vi "mqttClient_Viewer.vi"() -> ()   [LabVIEW 2019]
uses:
  <vilib>/LabVIEW Open Source Project/OpenSerializer JKI JSON/Serializer.JSON.lvclass
  C:/Program Files (x86)/National Instruments/LabVIEW 2019/vi.lib/LabVIEW Open Source Project/OpenSerializer/Serializer/Serializer.lvclass
  DUT/state -- cluster.ctl
  <vilib>/LabVIEW Open Source Project/MQTT Connection/MQTT_Base/Base Class/MQTT_Base.lvclass/MQTT_Base.ctl
  <vilib>/LabVIEW Open Source Project/MQTT Client/Client class/Client.lvclass/Client.ctl
  DUT/target -- cluster.ctl
  <vilib>/LabVIEW Open Source Project/MQTT Control Packets/Control Packets/ControlPacket/QualityOfService -- enum.ctl
  <vilib>/LabVIEW Open Source Project/MQTT Control Packets/Control Packets/ControlPacket/ControlPacket.lvclass/ControlPacket.ctl
  <vilib>/LabVIEW Open Source Project/MQTT Control Packets/Control Packets/CONNECT/ConnectFlags -- cluster.ctl
  <vilib>/LabVIEW Open Source Project/MQTT TCP Connection/MQTT_TCP/Connection/TCPConnection.lvclass
  C:/Program Files (x86)/National Instruments/LabVIEW 2019/vi.lib/LabVIEW Open Source Project/MQTT Connection/MQTT_Connection/Connection/Connection.lvclass
  <vilib>/LabVIEW Open Source Project/MQTT Client/Client class/Client.lvclass
  C:/Program Files (x86)/National Instruments/LabVIEW 2019/vi.lib/LabVIEW Open Source Project/MQTT Connection/MQTT_Base/Base Class/MQTT_Base.lvclass
  <vilib>/LabVIEW Open Source Project/OpenSerializer/Serializer.FlattenedString/Serializer.FlattenedString.lvclass
  <vilib>/LabVIEW Open Source Project/MQTT Control Packets/Control Packets/PUBLISH/PUBLISH.lvclass
  C:/Program Files (x86)/National Instruments/LabVIEW 2019/vi.lib/LabVIEW Open Source Project/MQTT Control Packets/Control Packets/ControlPacket/ControlPacket.lvclass
  <vilib>/LabVIEW Open Source Project/OpenSerializer/Serializer/Serializer.lvclass
  <vilib>/LabVIEW Open Source Project/MQTT Connection/MQTT_Base/Base Class/MQTT_Base.lvclass
  <vilib>/LabVIEW Open Source Project/MQTT Control Packets/Control Packets/CONNECT/CONNECT.lvclass
  <vilib>/LabVIEW Open Source Project/MQTT Control Packets/Control Packets/ControlPacket/ControlPacket.lvclass
panel:
  out "Incoming Messages":string
  in  "Connection":bool
  out "last error":errorcluster
  in  "setpoint":dbl format="%.1g"
  in  "enabled":bool
  out "Waveform Chart":cluster{"setpoint":dbl, "measured":dbl}(graph)
  # "Native LabVIEW MQTT Client (View)"
  # "G Open Source Project for LabVIEW\nhttps://github.com/LabVIEW-Open-Source/MQTT-Client"
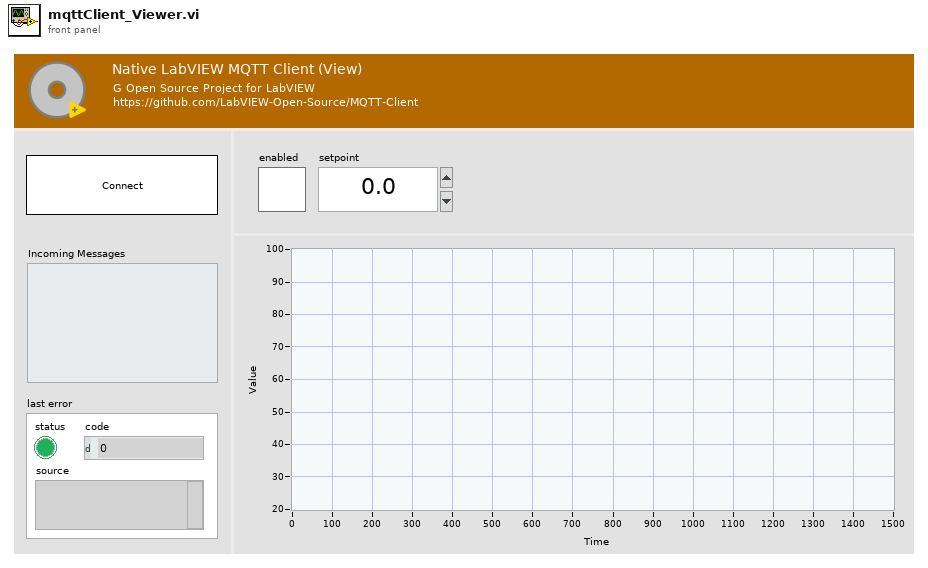
[diagram p1: front panel]
types:
  T1 = typedef "state -- cluster.ctl" = cluster{"enabled":bool, "setpoint":dbl, "measured":dbl}
  T2 = typedef "MQTT Client.lvlib/Client.lvclass/Public Events -- cluster.ctl" = cluster{"Connection Status":refnum<user-event>, "Connected":refnum<user-event>, "Application Message":refnum<user-event>}
  T3 = typedef "MQTT Base.lvlib/MQTT_Base.lvclass/Public Events -- cluster.ctl" = cluster{"Stop Event":refnum<user-event>, "Error Event":refnum<user-event>, "Inbound Message":refnum<user-event>}
  T4 = typedef "MQTT_Control_Packets.lvlib/ControlPacket.lvclass/QualityOfService -- enum.ctl" = enum16{"0 (At Most Once)", "1 (At Least Once)", "2 (Exactly Once)"}
  T5 = typedef "MQTT_Control_Packets.lvlib/CONNECT.lvclass/ConnectFlags -- cluster.ctl" = cluster{"Reserved":bool, "Clean Session":bool, "Will Flag":bool, "Will QoS 1":bool, "Will QoS 2":bool, "Will Retain":bool, "Password Flag":bool, "User Name Flag":bool}
  T6 = typedef "target -- cluster.ctl" = cluster{"enabled":bool, "setpoint":dbl}
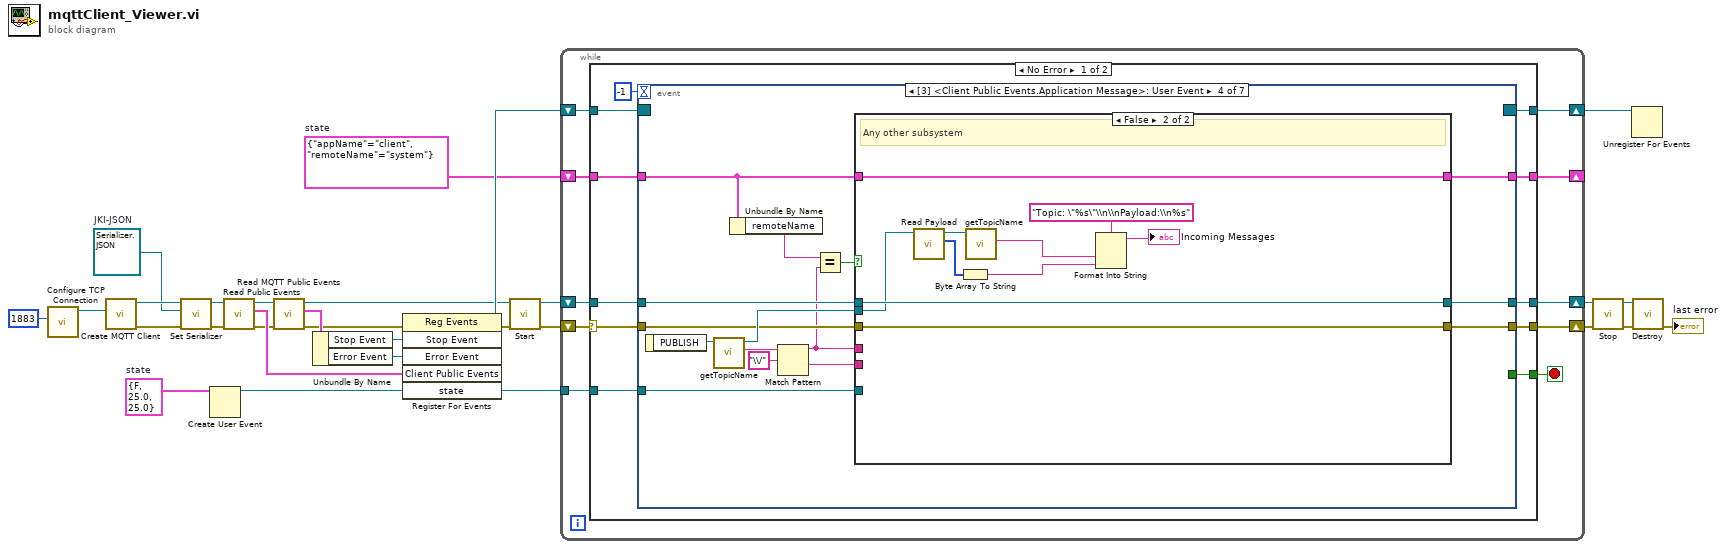
[diagram p0: block diagram]
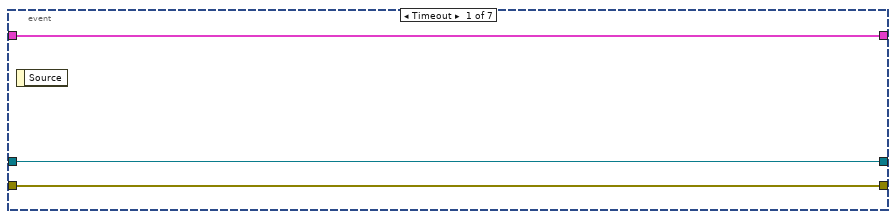
[diagram p2: hidden frame]
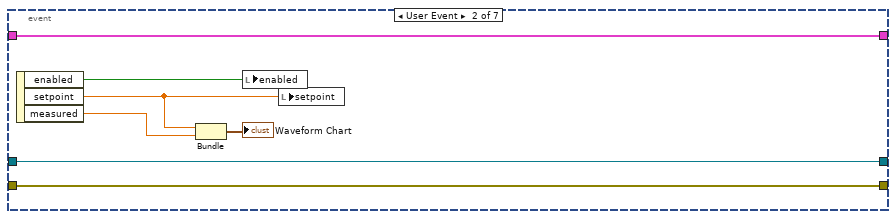
[diagram p3: hidden frame]
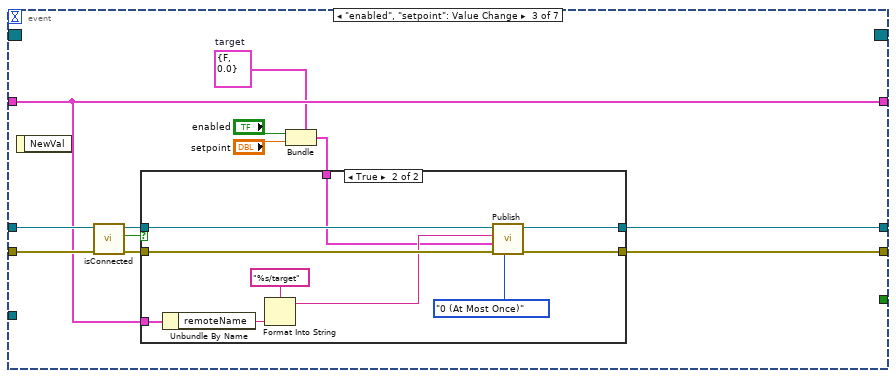
[diagram p4: hidden frame]
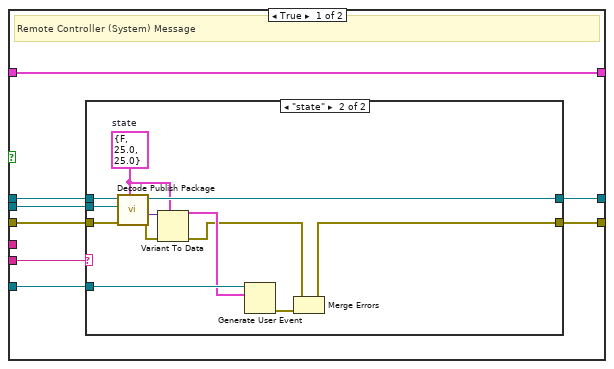
[diagram p6: hidden frame]
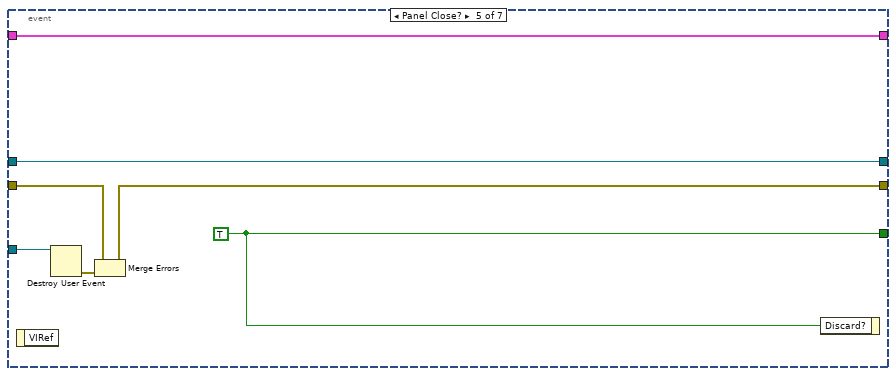
[diagram p8: hidden frame]
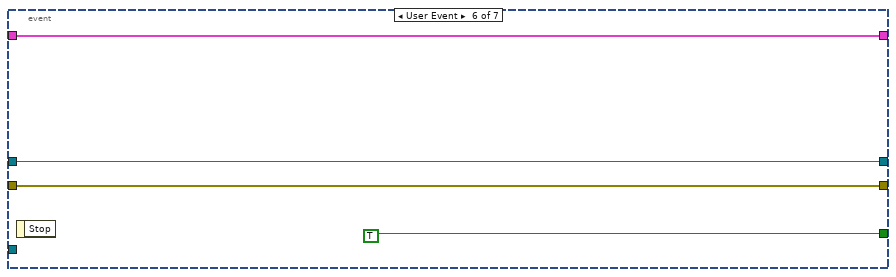
[diagram p9: hidden frame]
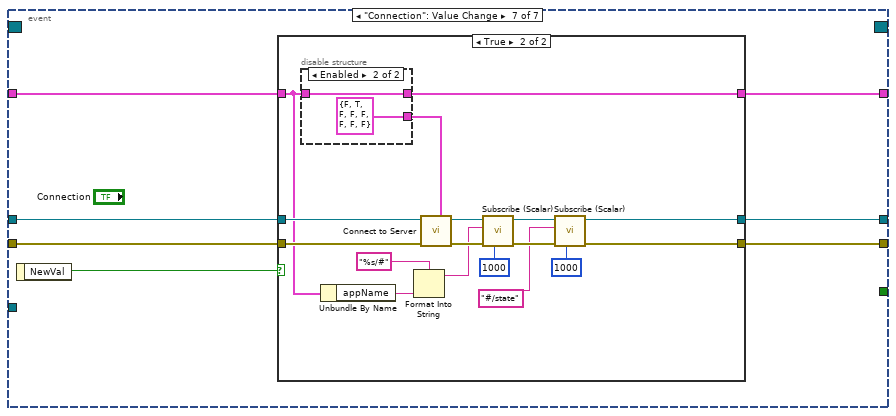
[diagram p10: hidden frame]
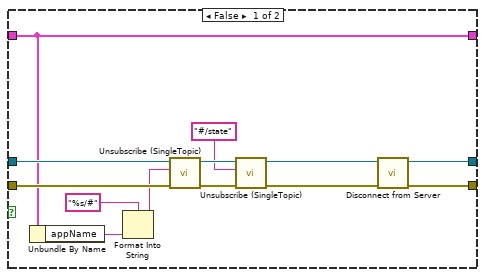
[diagram p11: hidden frame]
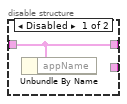
[diagram p12: hidden frame]
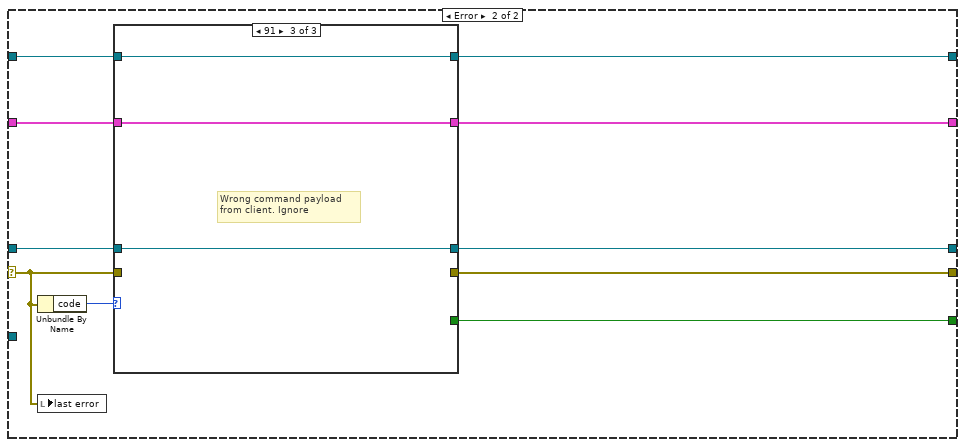
[diagram p13: hidden frame]
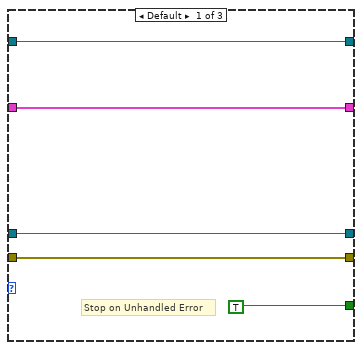
[diagram p14: hidden frame]
diagram:
  w2 = T1 {"enabled"=FALSE, "setpoint"=25.0, "measured"=25.0}  # state
  w3 = cluster{"appName":string, "remoteName":string} {"appName"="client", "remoteName"="system"}  # state
  w6 = refnum<class "Serializer.JSON.lvclass"> refnum  # JKI-JSON
  n1 = call <vilib>:"Configure TCP Connection.vi"("remote port (80)"=u16 1883) -> ("TCPConnection"=w11:refnum<class "TCPConnection.lvclass">)  [unwired: 9 in, 1 out]
  n2 = call <vilib>:"Create MQTT Client.vi"("Connection Configuration"=w11) -> ("error out"=w8:errorcluster, "Client out"=w10:refnum<class "Client.lvclass">)  [unwired: 9 in]
  n3 = call <vilib>:"Set Serializer.vi"("error in (no error)"=w8, "Serializer (default: Flattened String)"=w6, "MQTT_Base"=w10) -> ("error out"=w7:errorcluster, "MQTT_Base out"=w9:refnum<class "Client.lvclass">)  [unwired: 7 in]
  n4 = Create User Event(user event datatype=w2) -> (user event=w1:refnum<user-event>)  [unwired: 1 in, 1 out]
  n5 = call <vilib>:"Read Public Events.vi"("error in (no error)"=w7, "Client in"=w9) -> ("error out"=w13:errorcluster, "Client Public Events"=w15:T2, "Client out"=w12:refnum<class "Client.lvclass">)  [unwired: 7 in]
  n6 = call <vilib>:"Read MQTT Public Events.vi"("error in (no error)"=w13, "MQTT_Base in"=w12) -> ("error out"=w14:errorcluster, "MQTT Public Events"=w22:T3, "MQTT_Base out"=w17:refnum<class "Client.lvclass">)  [unwired: 7 in]
  n7 = Unbundle By Name(w22) -> ("Stop Event"=w20:refnum<user-event>, "Error Event"=w21:refnum<user-event>)
  n8 = register-events(error in=w14, w20, w21, w15, w1) -> (reference out=w18:refnum<event-registration>, error out=w16:errorcluster)  [unwired: 1 in]
  n9 = call <vilib>:"Start.vi"("error in (no error)"=w16, "MQTT_Base in"=w17) -> ("error out"=w4:errorcluster, "MQTT_Base out"=w5:refnum<class "Client.lvclass">)  [unwired: 7 in, 1 out]
  n10 = while {
    shift-right: [w37] -> w19
    shift-left: w18 -> [w38]
    shift-right: [w34] -> w24
    shift-left: w5 -> [w35]
    shift-right: [w36] -> w26
    shift-left: w4 -> [w32]
    shift-right: [w30] -> _
    shift-left: w3 -> [w31]
    tunnel: w1 -> [w29]
    stop <- w33 stop-if-true
    n11 = case shown="No Error" w32 {
      selector: w32 -> [w42 w185]
      tunnel: w38 -> [w49 w184]
      tunnel: [w48 w183] -> w37
      tunnel: [w47 w188] -> w36
      tunnel: w35 -> [w45 w189]
      tunnel: [w44 w191] -> w34
      tunnel: [w43 w187] -> w33
      tunnel: w31 -> [w41 w186]
      tunnel: [w40 w182] -> w30
      tunnel: w29 -> [w39 _]
      frame No Error {
        n12 = event shown="[3] <Client Public Events.Application Message>: User Event" {
          selector: w49 -> [_ _ _ _ _ _ _]
          dyn-events: [_ _ _ _ _ _ _] -> w48
          timeout: -1 -> [_ _ _ _ _ _ _]
          tunnel: w42 -> [w50 w57 w67 w95 w131 w141 w144]
          tunnel: [w50 w57 w61 w93 w132 w141 w145] -> w47
          tunnel: [_ _ _ _ w137 TRUE _] -> w43
          tunnel: w45 -> [w51 w58 w68 w96 w136 w139 w148]
          tunnel: [w51 w58 w62 w94 w136 w139 w146] -> w44
          tunnel: w41 -> [w52 w59 w66 w87 w135 w138 w142]
          tunnel: [w52 w59 w66 w92 w135 w138 w143] -> w40
          tunnel: w39 -> [_ _ _ w84 w134 _ _]
          event Timeout {
            n13 = event-data() -> ()  [unwired: 1 in, 1 out]
          }
          event User Event {
            n14 = event-data() -> ("enabled"=w55:bool, "setpoint"=w53:dbl, "measured"=w54:dbl)  [unwired: 1 in]
            n15 = Bundle("setpoint"=w53, "measured"=w54) -> (→"Waveform Chart":cluster{"setpoint":dbl, "measured":dbl})  [unwired: 1 in]
            n16 = local write "enabled"(w55) -> ()
            n17 = local write "setpoint"(w53) -> ()
          }
          event "enabled", "setpoint": Value Change {
            w60 = T6 {"enabled"=FALSE, "setpoint"=0.0}  # target
            n18 = event-data() -> ()  [unwired: 1 in, 1 out]
            n19 = call <vilib>:"isConnected.vi"("error in (no error)"=w67, "Client in"=w68) -> ("error out"=w71:errorcluster, "connected"=w69:bool, "Client out"=w70:refnum<class "Client.lvclass">)  [unwired: 7 in]
            n20 = Bundle(cluster=w60, "enabled"="enabled", "setpoint"="setpoint") -> (w63:T6)
            n21 = case shown="True" w69 {
              tunnel: [w73 w82] -> w62
              tunnel: [w72 w80] -> w61
              tunnel: w70 -> [w73 w83]
              tunnel: w71 -> [w72 w81]
              tunnel: w66 -> [_ w75]
              tunnel: w63 -> [_ w74]
              frame False {
              }
              frame True {
                n22 = Unbundle By Name(w75) -> ("remoteName"=w78:string)
                n23 = Format Into String(format string="%s/target" ("Topic Name (empty: Payload name)"), w78) -> (resulting string=w76:string)  [unwired: 2 in, 1 out]
                n24 = call <vilib>:"Publish.vi"("QoS"=QualityOfService_--_enum."0 (At Most Once)", "error in (no error)"=w81, "Payload"=w74, "Topic Name (empty: Payload name)"=w76, "Client in"=w83) -> ("error out"=w80:errorcluster, "Client out"=w82:refnum<class "Client.lvclass">)  [unwired: 4 in, 1 out]
              }
            }
          }
          event User Event {
            n25 = event-data() -> ("PUBLISH"=w98:refnum<class "PUBLISH.lvclass">)  [unwired: 1 in]
            n26 = call <vilib>:"getTopicName.vi"("PUBLISH in"=w98) -> ("Topic"=w90:string, "PUBLISH out"=w97:refnum<class "PUBLISH.lvclass">)  [unwired: 8 in, 1 out]
            n27 = Unbundle By Name(w87) -> ("remoteName"=w88:string)
            n28 = Match Pattern(string=w90, regular expression="\\/") -> (before substring=w86:string, after substring=w89:string)  [unwired: 1 in, 2 out]
            n29 = Equal?(x=w88, y=w86) -> (x = y?=w85:bool)
            n30 = case shown="False" w85 {
              tunnel: w97 -> [w103 w121]
              tunnel: w96 -> [w105 w129]
              tunnel: w95 -> [w104 w128]
              tunnel: [w102 w129] -> w94
              tunnel: [w101 w128] -> w93
              tunnel: w87 -> [w106 w130]
              tunnel: [w106 w130] -> w92
              tunnel: w89 -> [w100 _]
              tunnel: w86 -> [_ _]
              tunnel: w84 -> [w99 _]
              frame True {
                # "Remote Controller (System) Message"
                n31 = case shown="\"state\"" w100 {
                  tunnel: w105 -> [w108 w120]
                  tunnel: w104 -> [w107 w119]
                  tunnel: w103 -> [_ w118]
                  tunnel: [w108 w117] -> w102
                  tunnel: [w107 w109] -> w101
                  tunnel: w99 -> [_ w113]
                  frame Default {
                  }
                  frame "state" {
                    w114 = T1 {"enabled"=FALSE, "setpoint"=25.0, "measured"=25.0}  # state
                    n32 = call <vilib>:"Decode Publish Package.vi"("Type"=w114, "error in (no error)"=w119, "PUBLISH"=w118, "MQTT_Base in"=w120) -> ("error out"=w115:errorcluster, "Payload"=w116:variant, "MQTT_Base out"=w117:refnum<class "Client.lvclass">)  [unwired: 4 in, 1 out]
                    n33 = Variant To Data(error in=w115, type=w114, Variant=w116) -> (data=w112:T1, error out=w110:errorcluster)
                    n34 = Generate User Event(user event=w113, event data cluster=w112) -> (error out=w111:errorcluster)  [unwired: 2 in, 1 out]
                    n35 = Merge Errors(w110, w111) -> (w109:errorcluster)
                  }
                }
              }
              frame False {
                # "Any other subsystem"
                n36 = call <vilib>:"Read Payload.vi"("ControlPacket in"=w121) -> ("Payload"=w127:u8[], "ControlPacket out"=w126:refnum<class "PUBLISH.lvclass">)  [unwired: 9 in]
                n37 = Byte Array To String(unsigned byte array=w127) -> (string=w124:string)
                n38 = call <vilib>:"getTopicName.vi"("PUBLISH in"=w126) -> ("Topic"=w123:string)  [unwired: 8 in, 2 out]
                n39 = Format Into String(format string="Topic: \"%s\"\\n\\nPayload:\\n%s", w123, w124) -> (resulting string=→"Incoming Messages":string)  [unwired: 2 in, 1 out]
              }
            }
          }
          event Panel Close? {
            w137 = TRUE
            n40 = event-data() -> ()  [unwired: 1 in, 1 out]
            n41 = Destroy User Event(user event=w134) -> (error out=w133:errorcluster)  [unwired: 1 in]
            n42 = Merge Errors(w131, w133) -> (w132:errorcluster)
            n43 = event-data("Discard?"=w137) -> ()  [unwired: 1 in, 1 out]
          }
          event User Event {
            n44 = event-data() -> ()  [unwired: 1 in, 1 out]
          }
          event "Connection": Value Change {
            n45 = event-data() -> ("NewVal"=w147:bool)  [unwired: 1 in]
            n46 = case shown="True" w147 {
              tunnel: w148 -> [w159 w178]
              tunnel: [w161 w164] -> w146
              tunnel: [w160 w163] -> w145
              tunnel: w144 -> [w158 w177]
              tunnel: [w155 w176] -> w143
              tunnel: w142 -> [w155 w170]
              frame False {
                n47 = Unbundle By Name(w155) -> ("appName"=w157:string)
                n48 = Format Into String(format string="%s/#" ("Topic Name (empty: Payload name)"), w157) -> (resulting string=w154:string)  [unwired: 2 in, 1 out]
                n49 = call <vilib>:"Unsubscribe (SingleTopic).vi"("error in (no error)"=w158, "Topic Filter"=w154, "MQTT_Base in"=w159) -> ("error out"=w153:errorcluster, "MQTT_Base out"=w152:refnum<class "Client.lvclass">)  [unwired: 6 in, 1 out]
                n50 = call <vilib>:"Unsubscribe (SingleTopic).vi"("error in (no error)"=w153, "Topic Filter"="#/state" ("Topic Name (empty: Payload name)"), "MQTT_Base in"=w152) -> ("error out"=w150:errorcluster, "MQTT_Base out"=w151:refnum<class "Client.lvclass">)  [unwired: 6 in, 1 out]
                n51 = call <vilib>:"Disconnect from Server.vi"("error in (no error)"=w150, "Client in"=w151) -> ("error out"=w160:errorcluster, "Client out"=w161:refnum<class "Client.lvclass">)  [unwired: 7 in, 1 out]
              }
              frame True {
                n52 = disable-structure shown="Enabled" {
                  disable-tunnel: w170 -> [w179 w181]
                  disable-tunnel: [w179 w181] -> w176
                  disable-tunnel: [_ T5 {"Reserved"=FALSE, "Clean Session"=TRUE, "Will Flag"=FALSE, "Will QoS 1"=FALSE, "Will QoS 2"=FALSE, "Will Retain"=FALSE, "Password Flag"=FALSE, "User Name Flag"=FALSE} ("Connect Flags")] -> w175
                  frame Disabled {
                    n53 = Unbundle By Name(w179) -> ()  [unwired: 1 out]
                  }
                  frame Enabled {
                  }
                }
                n54 = Unbundle By Name(w170) -> ("appName"=w171:string)
                n55 = Format Into String(format string="%s/#" ("Topic Name (empty: Payload name)"), w171) -> (resulting string=w168:string)  [unwired: 2 in, 1 out]
                n56 = call <vilib>:"Connect to Server.vi"("Connect Flags"=w175, "error in (no error)"=w177, "Client in"=w178) -> ("error out"=w172:errorcluster, "Client out"=w173:refnum<class "Client.lvclass">)  [unwired: 5 in, 2 out]
                n57 = call <vilib>:"Subscribe (Scalar).vi"("timeout (1000ms)"=1000 ("timeout (100ms)"), "error in (no error)"=w172, "Topic Filter"=w168, "Client in"=w173) -> ("error out"=w165:errorcluster, "Client out"=w166:refnum<class "Client.lvclass">)  [unwired: 5 in, 1 out]
                n58 = call <vilib>:"Subscribe (Scalar).vi"("timeout (1000ms)"=1000 ("timeout (100ms)"), "error in (no error)"=w165, "Topic Filter"="#/state" ("Topic Name (empty: Payload name)"), "Client in"=w166) -> ("error out"=w163:errorcluster, "Client out"=w164:refnum<class "Client.lvclass">)  [unwired: 5 in, 1 out]
              }
            }
          }
        }
      }
      frame Error {
        n59 = Unbundle By Name(w185) -> ("code"=w190:i32)
        n60 = local write "last error"(w185) -> ()
        n61 = case shown="91" w190 {
          tunnel: w189 -> [w196 w199 w202]
          tunnel: [w196 w199 w202] -> w191
          tunnel: w185 -> [w195 _ _]
          tunnel: [w195 _ _] -> w188
          tunnel: [TRUE _ _] -> w187
          tunnel: w186 -> [w192 w197 w200]
          tunnel: w184 -> [w193 w198 w201]
          tunnel: [w193 w198 w201] -> w183
          tunnel: [w192 w197 w200] -> w182
          frame Default {
            # "Stop on Unhandled Error"
          }
          frame 56, 66 {
            # "Disconnected"
          }
          frame 91 {
            # "Wrong command payload\nfrom client. Ignore"
          }
        }
      }
    }
  }
  n62 = call <vilib>:"Stop.vi"("error in (no error)"=w26, "MQTT_Base in"=w24) -> ("error out"=w25:errorcluster, "MQTT_Base out"=w23:refnum<class "Client.lvclass">)  [unwired: 7 in, 1 out]
  n63 = Unregister For Events(event registration refnum=w19) -> ()  [unwired: 1 in, 1 out]
  n64 = call <vilib>:"Destroy.vi"("error in (no error)"=w25, "MQTT_Base in"=w23) -> ("error out"=→"last error":errorcluster)  [unwired: 8 in, 1 out]
